vi "ASIC_Selecor canal Sumador (Mega Pija).vi"(7 "Espera acceso USB":u32, 8 "error in":errorcluster, 9 "Sumador":u8, 10 "Canal":u8, 11 "ftHandle_in":u32) -> (0 "error out":errorcluster, 1 "Reg 100":u16 format="%04x", 2 "Reg 101":u16 format="%04x", 3 "ftHandle_out":u32)   [LabVIEW 2009]
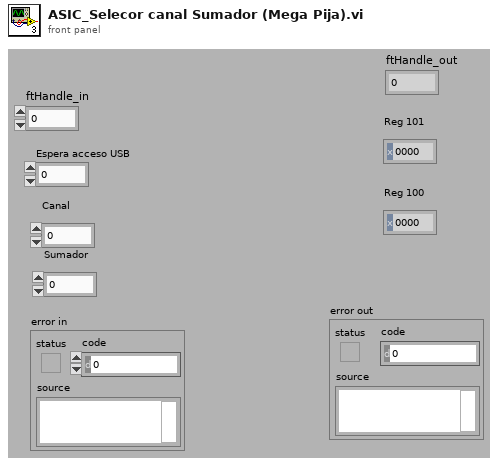
[diagram p1: front panel]
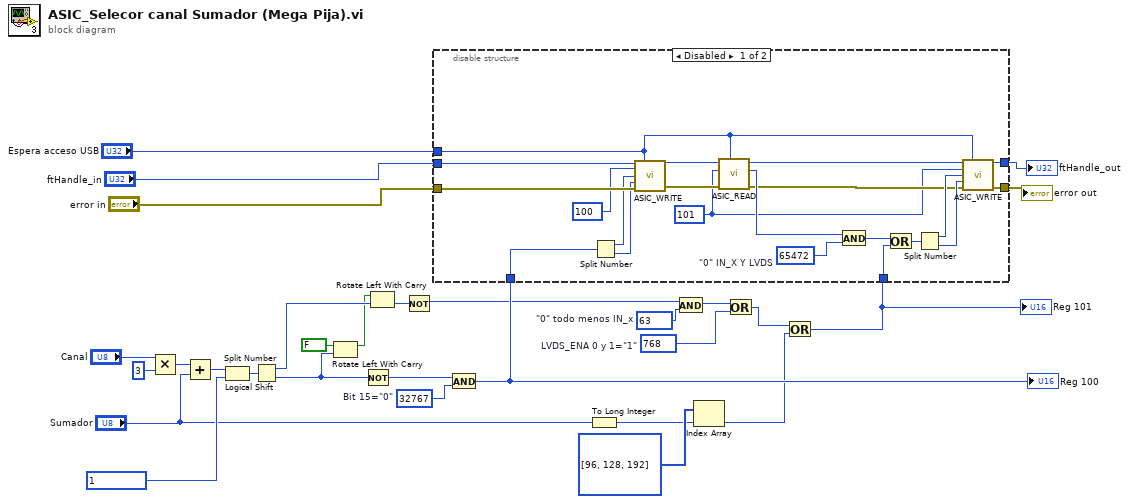
[diagram p0: block diagram]
diagram:
  w7 = u16 63  # "0" todo menos IN_x
  w17 = u16 768  # LVDS_ENA 0 y 1="1"
  w23 = u16 32767  # Bit 15="0"
  n1 = Multiply(x="Canal", y=u8 3 ("x")) -> (x*y=w26:u8)
  n2 = Add(x=w26, y="Sumador") -> (x+y=w25:u8)
  n3 = Logical Shift(y=w25, x=u32 1 ("x << y")) -> (x << y=w24:u32)
  n4 = Split Number(x=w24) -> (hi(x)=w20:u16, lo(x)=w22:u16)
  n5 = Rotate Left With Carry(2:w22, 3:FALSE ("carry")) -> (1:w19:bool)  [unwired: 1 out]
  n6 = Not(x=w22) -> (.not. x?=w16:u16)
  n7 = Rotate Left With Carry(2:w20, 3:w19) -> (0:w18:u16)  [unwired: 1 out]
  n8 = Not(x=w18) -> (.not. x?=w8:u16)
  n9 = And(x=w16, y=w23) -> (x .and. y?=w13:u16)
  "Reg 100" <- w13
  n10 = To Long Integer(number="Sumador") -> (32bit integer=w2:i32)
  n11 = And(x=w8, y=w7) -> (x .and. y?=w9:u16)
  n12 = Index Array(array=u16[] [96, 128, 192], index=w2) -> (element=w3:u16)
  n13 = Or(x=w9, y=w17) -> (x .or. y?=w6:u16)
  n14 = Or(x=w6, y=w3) -> (x .or. y?=w1:u16)
  "Reg 101" <- w1
  n15 = disable-structure shown="Disabled" {
    disable-tunnel: "ftHandle_in" -> [w50 _]
    disable-tunnel: "error in" -> [w49 _]
    disable-tunnel: w13 -> [w45 _]
    disable-tunnel: "Espera acceso USB" -> [w34 _]
    disable-tunnel: [w33 _] -> w11
    disable-tunnel: [w32 _] -> w10
    disable-tunnel: w1 -> [w30 _]
    frame #0 {
      w41 = u16 65472  # "0" IN_X Y LVDS
      w31 = u8 101 ("Direccion Registro Asic")
      n16 = Split Number(x=w45) -> (hi(x)=w47:u8, lo(x)=w46:u8)
      n17 = call "ASIC_WRITE.vi"("ftHandle_in"=w50, "Espera acceso USB"=w34, "Direccion Registro Asic"=u8 100, "Byte Alto"=w47, "Byte Bajo"=w46, "error in"=w49) -> ("ftHandle_out"=w44:u32, "error out"=w43:errorcluster)  [unwired: 8 in]
      n18 = call "ASIC_READ.vi"("Espera acceso USB"=w34, "error in"=w43, "Direccion Registro Asic"=w31, "ftHandle_in"=w44) -> ("error out"=w36:errorcluster, "Valor Asic"=w42:u16, "ftHandle_out"=w35:u32)  [unwired: 5 in]
      n19 = And(x=w42, y=w41) -> (x .and. y?=w40:u16)
      n20 = Or(x=w40, y=w30) -> (x .or. y?=w39:u16)
      n21 = Split Number(x=w39) -> (hi(x)=w38:u8, lo(x)=w37:u8)
      n22 = call "ASIC_WRITE.vi"("ftHandle_in"=w35, "Espera acceso USB"=w34, "Direccion Registro Asic"=w31, "Byte Alto"=w38, "Byte Bajo"=w37, "error in"=w36) -> ("ftHandle_out"=w33:u32, "error out"=w32:errorcluster)  [unwired: 8 in]
    }
    frame #1 {
    }
  }
  "ftHandle_out" <- w11
  "error out" <- w10
